vi "SCMP - Write Engineering Data to File.vi"(8 "error in":errorcluster, 9 "Temp Data":dbl[](array[numeric]), 10 "mesage":string, 11 "Base SCMP Log File Folder":path=path "C:/SCMP Logs") -> (0 "error out":errorcluster, 2 "Today's SCMP folder":path, 3 "first call":bool, 5 "Today's SCMP Engineering File":path)   [LabVIEW 2014]
doc: "This vi create or open file, which is save in format YYYYMMDD.txt. In this file are logs from CoMP-S Main program."
panel:
  in  "SCMP Eng File (\"static\")":path
  out "spreadsheet string":string
  out "Recent Log":string="\r"
  out "date/time string":string
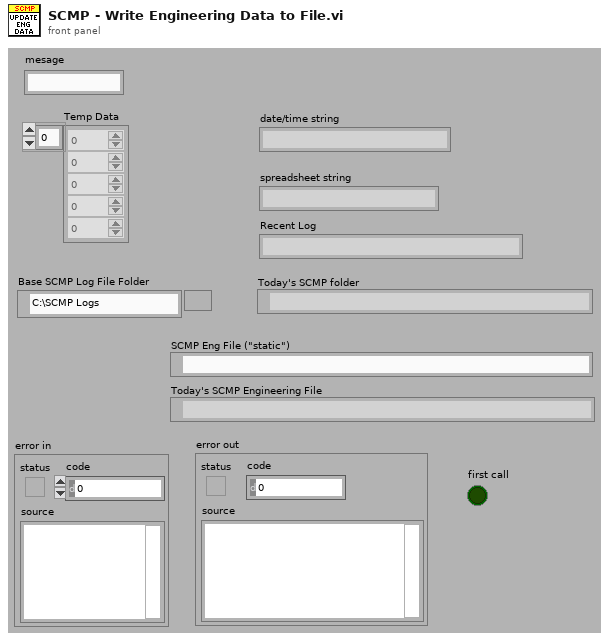
[diagram p1: front panel]
types:
  T1 = enum16{"open", "replace", "create", "open or create", "replace or create", "replace or create with confirmation"}
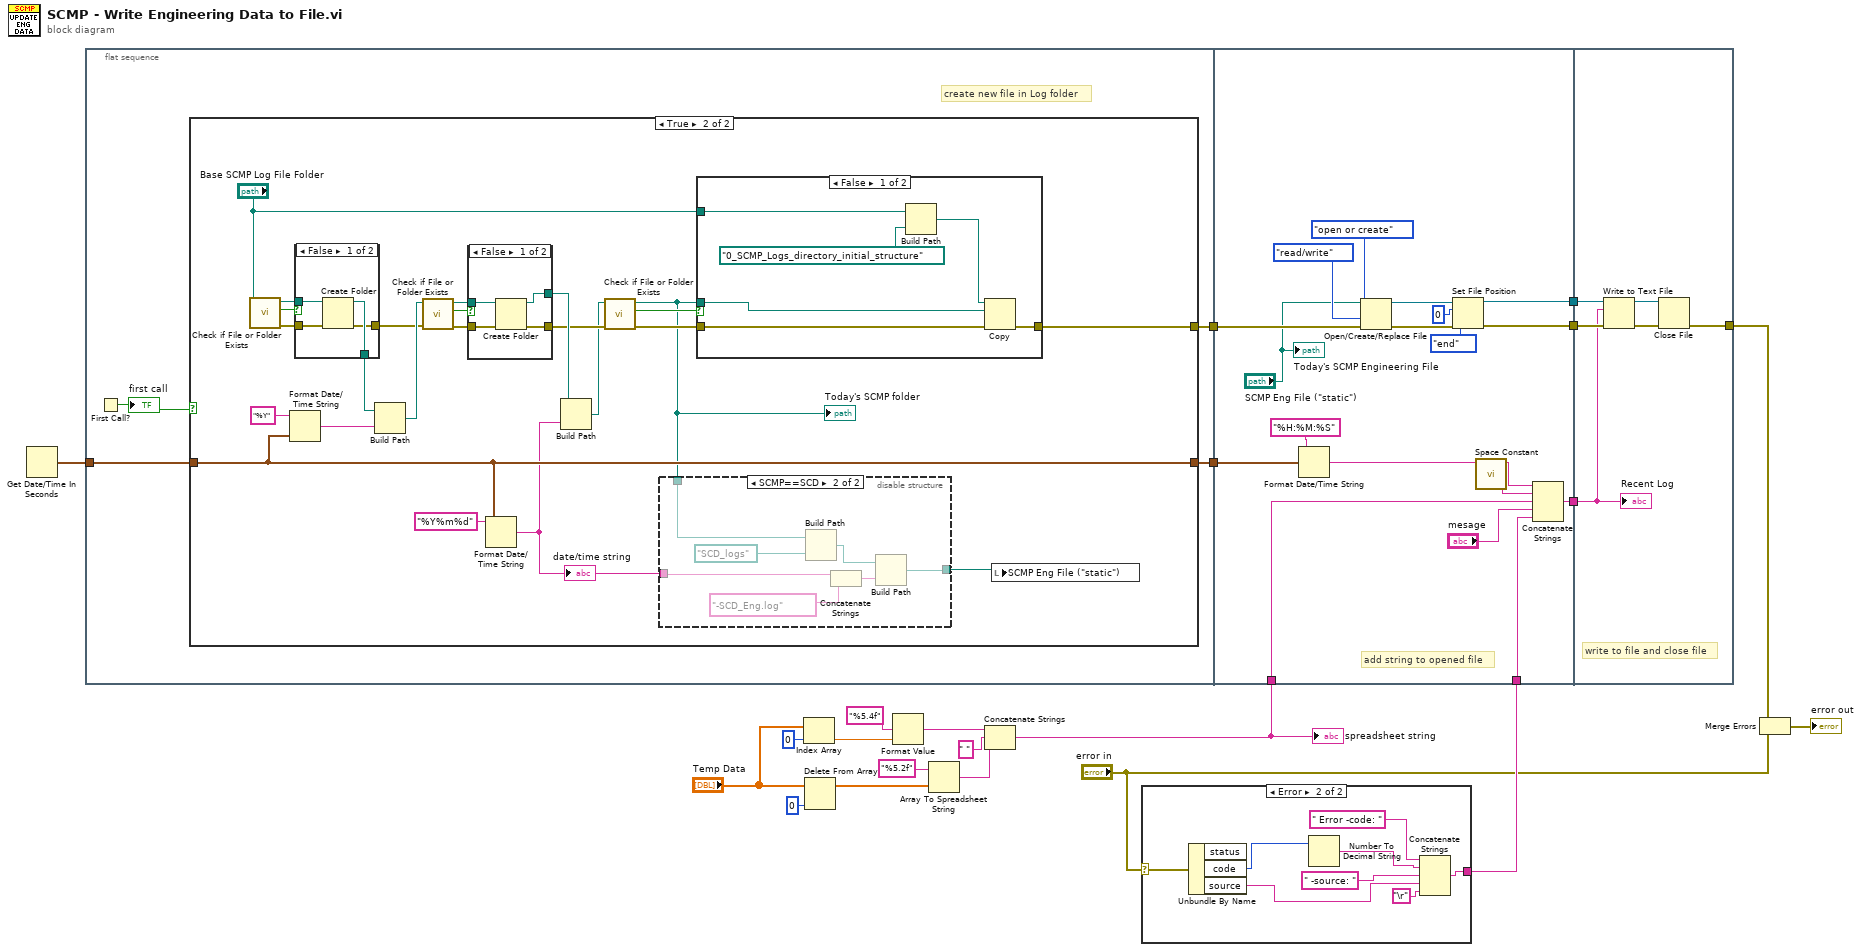
[diagram p0: block diagram]
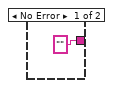
[diagram p2: hidden frame]
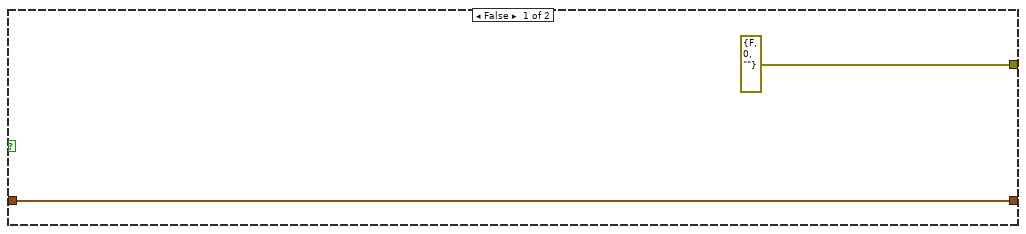
[diagram p3: hidden frame]
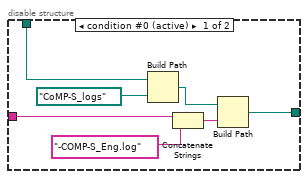
[diagram p4: hidden frame]
diagram:
  n1 = Get Date/Time In Seconds() -> (seconds since 1Jan1904=w3:timestamp)
  n2 = flat-sequence {
    tunnel: w3 -> [w25]
    tunnel: [w24] -> w2
    tunnel: [w22] -> w1
    tunnel: [w97] -> w21
    tunnel: [w91] -> w20
    tunnel: w13 -> [w95]
    tunnel: [w92] -> w18
    tunnel: w15 -> [w86]
    tunnel: w2 -> [w85]
    tunnel: w1 -> [w87]
    tunnel: w21 -> [w102]
    tunnel: w20 -> [w105]
    tunnel: w18 -> [w104]
    tunnel: [w103] -> w16
    frame #0 {
      # "create new file in Log folder"
      n3 = First Call?() -> (First Call?: T/F=w23:bool)
      "first call" <- w23
      n4 = case shown="True" w23 {
        tunnel: w25 -> [w26 w32]
        tunnel: [errorcluster {"status"=FALSE, "code"=0, "source"=""} ("error out") w30] -> w24
        tunnel: [w26 w32] -> w22
        frame False {
        }
        frame True {
          n5 = call <vilib>:"Check if File or Folder Exists.vi"("path"="Base SCMP Log File Folder") -> ("error out"=w39:errorcluster, "file or folder exists?"=w49:bool, "dup path"=w48:path)  [unwired: 8 in]
          n6 = Format Date/Time String(time format string (%c)="%Y", seconds (now)=w32) -> (date/time string=w46:string)  [unwired: 1 in]
          n7 = case shown="False" w49 {
            tunnel: w48 -> [w81 w83]
            tunnel: [w80 w83] -> w45
            tunnel: [w79 w82] -> w41
            tunnel: w39 -> [w78 w82]
            frame False {
              n8 = Create Folder(path (use dialog)=w81, error in=w78) -> (created path=w80:path, error out=w79:errorcluster)  [unwired: 1 in, 1 out]
            }
            frame True {
            }
          }
          n9 = Build Path(base path=w45, name or relative path=w46) -> (appended path=w42:path)
          n10 = call <vilib>:"Check if File or Folder Exists.vi"("error in (no error)"=w41, "path"=w42) -> ("error out"=w40:errorcluster, "file or folder exists?"=w44:bool, "dup path"=w43:path)  [unwired: 7 in]
          n11 = case shown="False" w44 {
            tunnel: w43 -> [w75 w76]
            tunnel: w40 -> [w74 w77]
            tunnel: [w73 w77] -> w35
            tunnel: [w72 w76] -> w36
            frame False {
              n12 = Create Folder(path (use dialog)=w75, error in=w74) -> (created path=w72:path, error out=w73:errorcluster)  [unwired: 1 in, 1 out]
            }
            frame True {
            }
          }
          n13 = Format Date/Time String(time format string (%c)="%Y%m%d", seconds (now)=w32) -> (date/time string=w29:string)  [unwired: 1 in]
          "date/time string" <- w29
          n14 = Build Path(base path=w36, name or relative path=w29) -> (appended path=w34:path)
          n15 = call <vilib>:"Check if File or Folder Exists.vi"("error in (no error)"=w35, "path"=w34) -> ("error out"=w38:errorcluster, "file or folder exists?"=w37:bool, "dup path"=w28:path)  [unwired: 7 in]
          "Today's SCMP folder" <- w28
          n16 = disable-structure shown="SCMP==SCD" {
            disable-tunnel: [w56 w60] -> w33
            disable-tunnel: w29 -> [w53 w59]
            disable-tunnel: w28 -> [w51 w58]
            frame condition #0 (active) {
              n17 = Build Path(base path=w51, name or relative path=path "CoMP-S_logs") -> (appended path=w54:path)
              n18 = Concatenate Strings(w53, "-COMP-S_Eng.log" ("string")) -> (w57:string)
              n19 = Build Path(base path=w54, name or relative path=w57) -> (appended path=w56:path)
            }
            frame condition #1 {
              n20 = Build Path(base path=w58, name or relative path=path "SCD_logs") -> (appended path=w62:path)
              n21 = Concatenate Strings(w59, "-SCD_Eng.log" ("string")) -> (w64:string)
              n22 = Build Path(base path=w62, name or relative path=w64) -> (appended path=w60:path)
            }
          }
          n23 = case shown="False" w37 {
            tunnel: w28 -> [w65 _]
            tunnel: w38 -> [w67 w71]
            tunnel: "Base SCMP Log File Folder" -> [w70 _]
            tunnel: [w66 w71] -> w30
            frame False {
              n24 = Build Path(base path=w70, name or relative path=path "0_SCMP_Logs_directory_initial_structure") -> (appended path=w68:path)
              n25 = Copy(8:w67, 10:w65, 11:w68) -> (0:w66:errorcluster)  [unwired: 2 in, 2 out]
            }
            frame True {
            }
          }
          n26 = local write "SCMP Eng File (\"static\")"(w33) -> ()
        }
      }
    }
    frame #1 {
      # "add string to opened file"
      n27 = Format Date/Time String(time format string (%c)="%H:%M:%S", seconds (now)=w87) -> (date/time string=w99:string)  [unwired: 1 in]
      n28 = Open/Create/Replace File(file path (use dialog)="SCMP Eng File (\"static\")", error in=w85, operation (0:open)=T1."open or create", access (0:read/write)=enum16{"read/write", "read-only", "write-only"}."read/write") -> (refnum out=w93:refnum<file>, error out=w94:errorcluster)  [unwired: 3 out]
      n29 = Set File Position(offset (in bytes) (0)=i64 0, refnum=w93, from (0:start)=enum16{"start", "end", "current"}."end", error in=w94) -> (refnum out=w91:refnum<file>, error out=w92:errorcluster)
      n30 = call <vilib>:"Space Constant.vi"() -> ("String"=w98:string)
      n31 = Concatenate Strings(w99, w98, w95, "mesage", w86) -> (w97:string)
      "Today's SCMP Engineering File" <- "SCMP Eng File (\"static\")"
    }
    frame #2 {
      # "write to file and close file"
      n32 = Write to Text File(file (use dialog)=w105, text=w102, error in=w104) -> (refnum out=w106:refnum<file>, error out=w107:errorcluster)  [unwired: 1 in, 1 out]
      n33 = Close File(refnum=w106, error in=w107) -> (error out=w103:errorcluster)  [unwired: 1 out]
      "Recent Log" <- w102
    }
  }
  n34 = Index Array(array="Temp Data", index=0) -> (element=w8:dbl)
  n35 = Delete From Array(array="Temp Data", index=0) -> (array with subset deleted=w11:dbl[])  [unwired: 1 in, 1 out]
  n36 = Format Value(format string="%5.4f", value (0)=w8) -> (output string=w6:string)  [unwired: 1 in]
  n37 = Array To Spreadsheet String(array=w11, 3:"%5.2f" ("format string")) -> (spreadsheet string=w5:string)  [unwired: 1 in]
  n38 = Concatenate Strings(w6, " " ("string"), w5) -> (w13:string)
  "spreadsheet string" <- w13
  n39 = case shown="Error" "error in" {
    selector: "error in" -> [_ w113]
    tunnel: ["" w110] -> w15
    frame No Error {
    }
    frame Error {
      n40 = Unbundle By Name(w113) -> ("code"=w112:i32, "source"=w111:string)  [unwired: 1 out]
      n41 = Number To Decimal String(number=w112) -> (decimal integer string=w116:string)  [unwired: 1 in]
      n42 = Concatenate Strings(" Error -code: ", w116, " -source: ", w111, "\r") -> (w110:string)
    }
  }
  n43 = Merge Errors(w16, "error in") -> (→"error out":errorcluster)
